vi "Get Voltage Resolution.vi"(11 "channel":i8) -> (3 "function return":dbl)   [LabVIEW 2021, in "vmmso.lvlib"]
doc: "DLL_API double WINAPI GetVoltageResolution(char channel);"
uses:
  vmmso.lvlib
  vmmso.dll
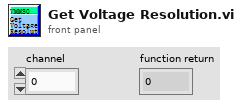
[diagram p1: front panel]
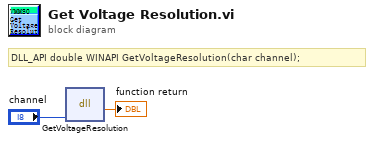
[diagram p0: block diagram]
diagram:
  # "DLL_API double WINAPI GetVoltageResolution(char channel);"
  n1 = dll-call lib="D:/labviewdemo/LabviewDemo 21/vmmso/vmmso.*" fn="GetVoltageResolution"("channel"="channel") -> (→"function return":dbl)  [unwired: 4 in, 2 out]
